vi "Assign values from string to axes_C-887.vi"(0 "System no.":i32=1 min=1 max=4 step=1, 2 "Queried axes":string[](array[string]), 3 "All axes queried?":bool, 4 "Input String":string, 5 "error in":errorcluster, 6 "Axes related?":bool=TRUE) -> (14 "Values":dbl[](array[numeric]) format="%.6f", 15 "Strings":string[](array[string]), 16 "Queried axes out":string[](array[string]), 19 "error out":errorcluster)   [LabVIEW 2020]
doc: "This VI assigns numerical values and/or single lines from input string to queried axes. If All axes is TRUE, connected axes are read from Global2.vi and displayed on the front panel for assignment."
panel:
  # "This vi assigns values and/or single lines from input string to queried axes. If \"All axes\" is true, connected axes are read from Global2.vi"
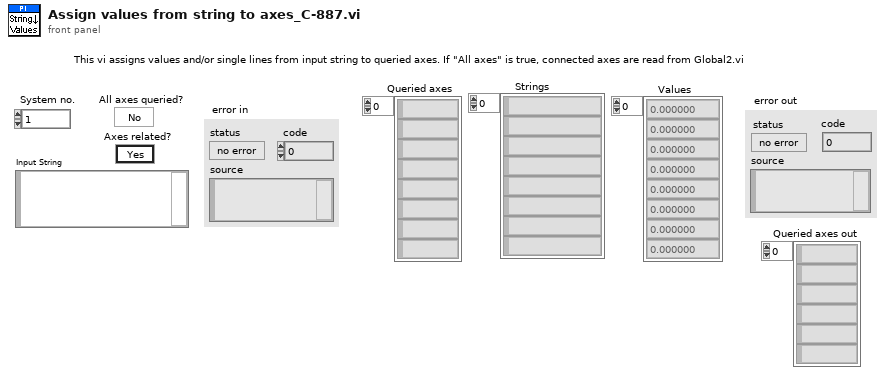
[diagram p1: front panel]
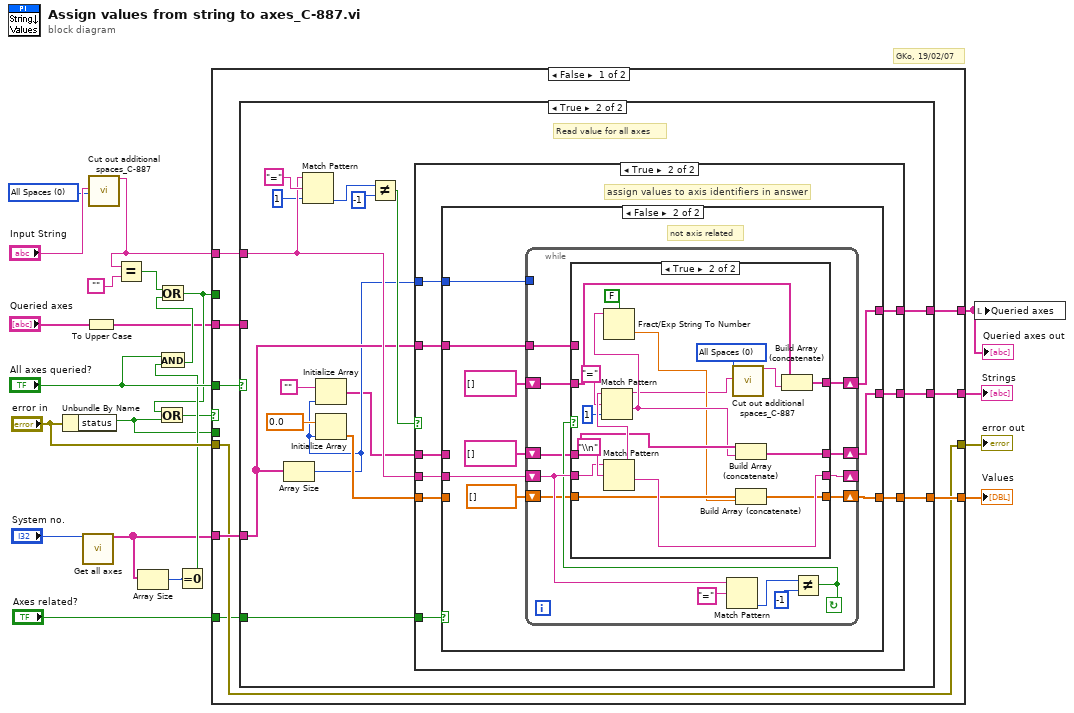
[diagram p0: block diagram]
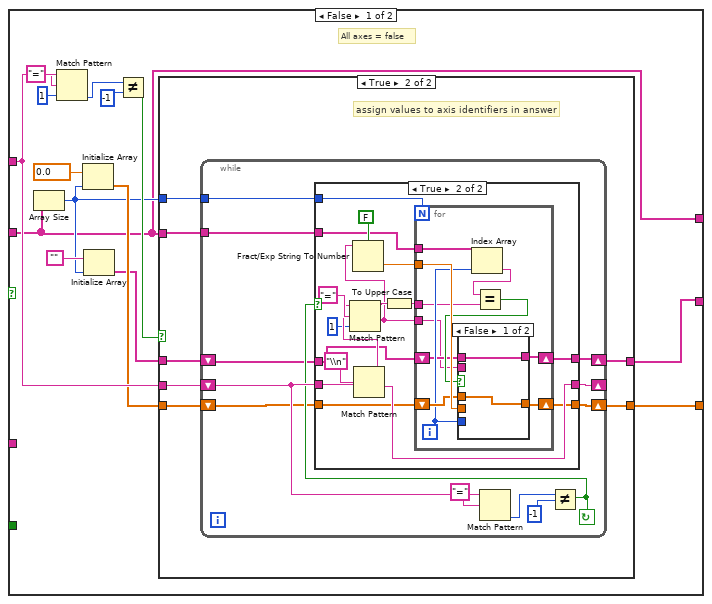
[diagram p2: hidden frame]
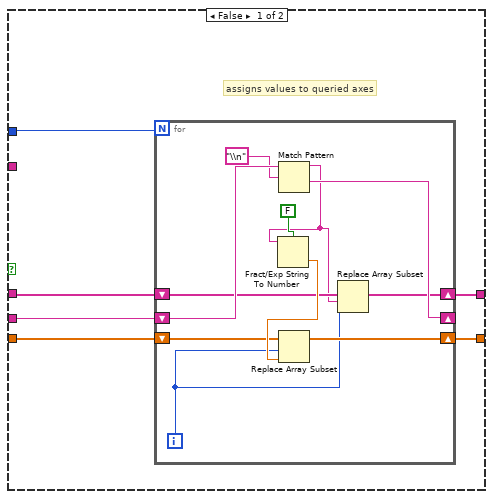
[diagram p3: hidden frame]
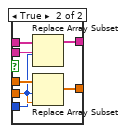
[diagram p5: hidden frame]
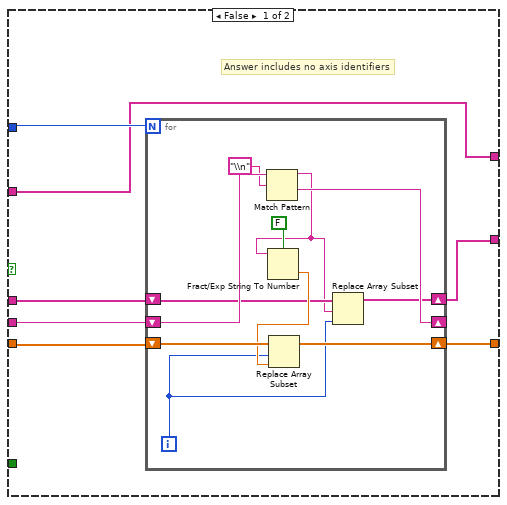
[diagram p6: hidden frame]
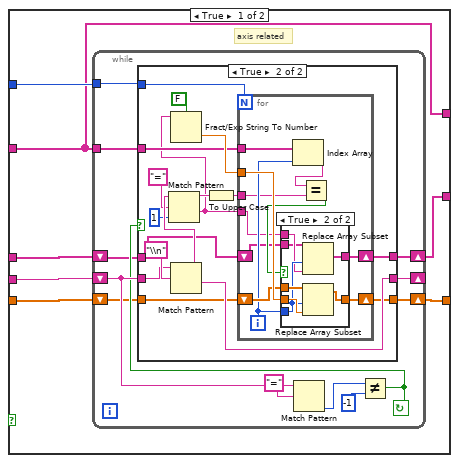
[diagram p7: hidden frame]
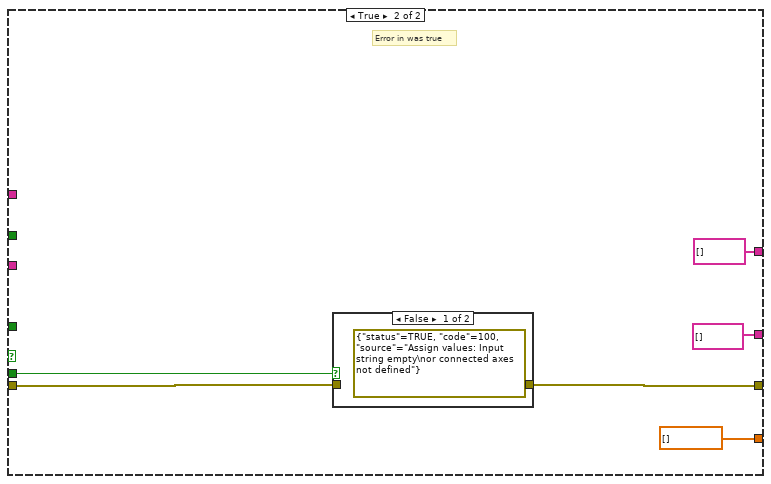
[diagram p11: hidden frame]
diagram:
  w4 = u16 0 items=["All Spaces", "Only if 1st char.", "Only if last char.", "Only if near \"=\""] ("Mode")
  # "GKo, 19/02/07"
  n1 = Unbundle By Name("error in") -> ("status"=w8:bool)
  n2 = call "Get all axes.vi"("System no."="System no.") -> ("Conn. Axes"=w6:string[])  [unwired: 18 out]
  n3 = To Upper Case(1:"Queried axes") -> (0:w10:string[])
  n4 = call "Cut out additional spaces_C-887.vi"("String"="Input String", "Mode"=w4) -> ("String out"=w3:string)  [unwired: 17 out]
  n5 = Equal?(x=w3, y="") -> (x = y?=w17:bool)
  n6 = Array Size(array=w6) -> (size(s)=w15:i32)
  n7 = Equal To 0?(x=w15) -> (x = 0?=w14:bool)
  n8 = And(x="All axes queried?", y=w14) -> (x .and. y?=w13:bool)
  n9 = Or(x=w17, y=w13) -> (x .or. y?=w11:bool)
  n10 = Or(x=w11, y=w8) -> (x .or. y?=w12:bool)
  n11 = case shown="False" w12 {
    tunnel: "All axes queried?" -> [w31 _]
    tunnel: w3 -> [w30 _]
    tunnel: [w29 dbl[] [] ("Step Size")] -> w22
    tunnel: w10 -> [w28 _]
    tunnel: w6 -> [w27 _]
    tunnel: [w26 w271] -> w19
    tunnel: "error in" -> [w26 w272]
    tunnel: w11 -> [_ _]
    tunnel: [w25 string[] []] -> w9
    tunnel: w8 -> [_ w269]
    tunnel: "Axes related?" -> [w24 _]
    tunnel: [w23 string[] [] ("Conn. Axes")] -> w1
    frame False {
      n12 = case shown="True" w31 {
        tunnel: w30 -> [w44 w133]
        tunnel: [w45 w137] -> w29
        tunnel: w28 -> [w32 _]
        tunnel: w27 -> [_ w129]
        tunnel: [w34 w125] -> w25
        tunnel: w24 -> [_ w123]
        tunnel: [w32 w122] -> w23
        frame False {
          # "All axes = false"
          n13 = Array Size(array=w32) -> (size(s)=w36:i32)
          n14 = Match Pattern(string=w44, regular expression="=", offset (0)=1) -> (offset past match=w41:i32)  [unwired: 3 out]
          n15 = Initialize Array(0.0 ("Element Data"), w36) -> (w38:dbl[])
          n16 = Initialize Array("", w36) -> (w35:string[])
          n17 = Not Equal?(x=w41, y=-1) -> (x != y?=w40:bool)
          n18 = case shown="True" w40 {
            tunnel: [w51 w68] -> w45
            tunnel: w44 -> [w50 w69]
            tunnel: w32 -> [_ w67]
            tunnel: w38 -> [w49 w65]
            tunnel: w36 -> [w48 w66]
            tunnel: w35 -> [w47 w64]
            tunnel: [w46 w63] -> w34
            frame False {
              # "assigns values to queried axes"
              n19 = for {
                N: w48 -> [_]
                shift-right: [w56] -> w51
                shift-left: w49 -> [w57]
                shift-right: [w61] -> _
                shift-left: w50 -> [w62]
                shift-right: [w55] -> w46
                shift-left: w47 -> [w54]
                i -> [w53]
                n20 = Match Pattern(string=w62, regular expression="\\n") -> (before substring=w52:string, after substring=w61:string)  [unwired: 3 out]
                n21 = Fract/Exp String To Number(use system decimal point (T)=FALSE, string=w52) -> (number=w58:dbl)  [unwired: 3 out]
                n22 = Replace Array Subset(array=w57, new element=w58, index=w53) -> (w56:dbl[])
                n23 = Replace Array Subset(array=w54, new element=w52, index=w53) -> (w55:string[])
              }
            }
            frame True {
              # "assign values to axis identifiers in answer"
              n24 = while {
                shift-left: w64 -> [w70]
                shift-right: [w71] -> w63
                tunnel: w66 -> [w72]
                tunnel: w67 -> [w73]
                shift-left: w65 -> [w75]
                shift-right: [w74] -> w68
                shift-left: w69 -> [w78]
                shift-right: [w77] -> _
                stop <- w76 continue-if-true
                n25 = Match Pattern(string=w78, regular expression="=") -> (offset past match=w79:i32)  [unwired: 4 out]
                n26 = Not Equal?(x=w79, y=-1) -> (x != y?=w76:bool)
                n27 = case shown="True" w76 {
                  tunnel: w78 -> [w84 w100]
                  tunnel: [w84 w99] -> w77
                  tunnel: [w83 w97] -> w74
                  tunnel: w75 -> [w83 w98]
                  tunnel: w73 -> [_ w92]
                  tunnel: w72 -> [_ w90]
                  tunnel: [w82 w88] -> w71
                  tunnel: w70 -> [w82 w87]
                  frame False {
                  }
                  frame True {
                    n28 = Match Pattern(string=w100, regular expression="\\n") -> (before substring=w94:string, after substring=w99:string)  [unwired: 3 out]
                    n29 = Match Pattern(string=w94, regular expression="=", offset (0)=1) -> (before substring=w91:string, after substring=w89:string)  [unwired: 2 out]
                    n30 = Fract/Exp String To Number(use system decimal point (T)=FALSE, string=w89) -> (number=w93:dbl)  [unwired: 3 out]
                    n31 = To Upper Case(1:w91) -> (0:w85:string)
                    n32 = for {
                      N: w90 -> [_]
                      tunnel: w93 -> [w112]
                      shift-right: [w110] -> w97
                      shift-left: w98 -> [w111]
                      tunnel: w92 -> [w108]
                      tunnel: w85 -> [w106]
                      shift-right: [w103] -> w88
                      shift-left: w87 -> [w104]
                      tunnel: w89 -> [w102]
                      i -> [w109]
                      n33 = Index Array(array=w108, index=w109) -> (element=w107:string)
                      n34 = Equal?(x=w107, y=w106) -> (x = y?=w105:bool)
                      n35 = case shown="False" w105 {
                        tunnel: w112 -> [_ w121]
                        tunnel: w109 -> [_ w118]
                        tunnel: w111 -> [w114 w120]
                        tunnel: [w114 w119] -> w110
                        tunnel: w104 -> [w113 w117]
                        tunnel: [w113 w116] -> w103
                        tunnel: w102 -> [_ w115]
                        frame False {
                        }
                        frame True {
                          n36 = Replace Array Subset(array=w117, new element=w115, index=w118) -> (w116:string[])
                          n37 = Replace Array Subset(array=w120, new element=w121, index=w118) -> (w119:dbl[])
                        }
                      }
                    }
                  }
                }
              }
            }
          }
        }
        frame True {
          # "Read value for all axes"
          n38 = Array Size(array=w129) -> (size(s)=w128:i32)
          n39 = Match Pattern(string=w133, regular expression="=", offset (0)=1) -> (offset past match=w134:i32)  [unwired: 3 out]
          n40 = Initialize Array("", w128) -> (w127:string[])
          n41 = Initialize Array(0.0 ("Element Data"), w128) -> (w130:dbl[])
          n42 = Not Equal?(x=w134, y=-1) -> (x != y?=w132:bool)
          n43 = case shown="True" w132 {
            tunnel: [w144 w164] -> w137
            tunnel: w133 -> [w143 w163]
            tunnel: w129 -> [w138 w162]
            tunnel: w130 -> [w142 w161]
            tunnel: w128 -> [w141 w160]
            tunnel: w127 -> [w140 w159]
            tunnel: [w139 w158] -> w125
            tunnel: w123 -> [_ w157]
            tunnel: [w138 w156] -> w122
            frame False {
              # "Answer includes no axis identifiers"
              n44 = for {
                N: w141 -> [_]
                shift-right: [w151] -> w144
                shift-left: w142 -> [w153]
                shift-right: [w154] -> _
                shift-left: w143 -> [w155]
                shift-right: [w146] -> w139
                shift-left: w140 -> [w148]
                i -> [w147]
                n45 = Match Pattern(string=w155, regular expression="\\n") -> (before substring=w145:string, after substring=w154:string)  [unwired: 3 out]
                n46 = Fract/Exp String To Number(use system decimal point (T)=FALSE, string=w145) -> (number=w152:dbl)  [unwired: 3 out]
                n47 = Replace Array Subset(array=w153, new element=w152, index=w147) -> (w151:dbl[])
                n48 = Replace Array Subset(array=w148, new element=w145, index=w147) -> (w146:string[])
              }
            }
            frame True {
              # "assign values to axis identifiers in answer"
              n49 = case shown="False" w157 {
                tunnel: [w171 w232] -> w164
                tunnel: w163 -> [w170 w231]
                tunnel: w162 -> [w165 w230]
                tunnel: w161 -> [w169 _]
                tunnel: w160 -> [w168 w229]
                tunnel: w159 -> [w167 _]
                tunnel: [w166 w228] -> w158
                tunnel: [w165 w224] -> w156
                frame True {
                  # "axis related"
                  n50 = while {
                    shift-left: w167 -> [w173]
                    shift-right: [w172] -> w166
                    tunnel: w168 -> [w174]
                    tunnel: w165 -> [w175]
                    shift-left: w169 -> [w177]
                    shift-right: [w176] -> w171
                    shift-left: w170 -> [w180]
                    shift-right: [w179] -> _
                    stop <- w178 continue-if-true
                    n51 = Match Pattern(string=w180, regular expression="=") -> (offset past match=w181:i32)  [unwired: 4 out]
                    n52 = Not Equal?(x=w181, y=-1) -> (x != y?=w178:bool)
                    n53 = case shown="True" w178 {
                      tunnel: w180 -> [w186 w202]
                      tunnel: [w186 w201] -> w179
                      tunnel: [w185 w199] -> w176
                      tunnel: w177 -> [w185 w200]
                      tunnel: w175 -> [_ w193]
                      tunnel: w174 -> [_ w192]
                      tunnel: w173 -> [w184 w191]
                      tunnel: [w184 w190] -> w172
                      frame False {
                      }
                      frame True {
                        n54 = Match Pattern(string=w202, regular expression="\\n") -> (before substring=w198:string, after substring=w201:string)  [unwired: 3 out]
                        n55 = Match Pattern(string=w198, regular expression="=", offset (0)=1) -> (before substring=w196:string, after substring=w189:string)  [unwired: 2 out]
                        n56 = Fract/Exp String To Number(use system decimal point (T)=FALSE, string=w189) -> (number=w195:dbl)  [unwired: 3 out]
                        n57 = To Upper Case(1:w196) -> (0:w187:string)
                        n58 = for {
                          N: w192 -> [_]
                          tunnel: w187 -> [w208]
                          tunnel: w195 -> [w214]
                          shift-right: [w212] -> w199
                          shift-left: w200 -> [w213]
                          tunnel: w193 -> [w211]
                          shift-right: [w206] -> w190
                          shift-left: w191 -> [w204]
                          tunnel: w189 -> [w205]
                          i -> [w210]
                          n59 = Index Array(array=w211, index=w210) -> (element=w209:string)
                          n60 = Equal?(x=w209, y=w208) -> (x = y?=w207:bool)
                          n61 = case shown="True" w207 {
                            tunnel: w214 -> [_ w223]
                            tunnel: w210 -> [_ w220]
                            tunnel: w213 -> [w216 w222]
                            tunnel: [w216 w221] -> w212
                            tunnel: [w215 w219] -> w206
                            tunnel: w205 -> [_ w218]
                            tunnel: w204 -> [w215 w217]
                            frame False {
                            }
                            frame True {
                              n62 = Replace Array Subset(array=w217, new element=w218, index=w220) -> (w219:string[])
                              n63 = Replace Array Subset(array=w222, new element=w223, index=w220) -> (w221:dbl[])
                            }
                          }
                        }
                      }
                    }
                  }
                }
                frame False {
                  # "not axis related"
                  n64 = while {
                    shift-left: string[] [] -> [w236]
                    shift-right: [w235] -> w228
                    tunnel: w229 -> [_]
                    tunnel: w230 -> [w237]
                    shift-left: dbl[] [] -> [w239]
                    shift-right: [w238] -> w232
                    shift-left: w231 -> [w242]
                    shift-right: [w241] -> _
                    shift-right: [w234] -> w224
                    shift-left: string[] [] -> [w233]
                    stop <- w240 continue-if-true
                    n65 = Match Pattern(string=w242, regular expression="=") -> (offset past match=w243:i32)  [unwired: 4 out]
                    n66 = Not Equal?(x=w243, y=-1) -> (x != y?=w240:bool)
                    n67 = case shown="True" w240 {
                      tunnel: w242 -> [w249 w266]
                      tunnel: [w249 w265] -> w241
                      tunnel: [w248 w263] -> w238
                      tunnel: w239 -> [w248 w264]
                      tunnel: w237 -> [_ _]
                      tunnel: w236 -> [w247 w259]
                      tunnel: [w247 w258] -> w235
                      tunnel: [w246 w251] -> w234
                      tunnel: w233 -> [w246 w250]
                      frame False {
                      }
                      frame True {
                        w253 = u16 0 items=["All Spaces", "Only if 1st char.", "Only if last char.", "Only if near \"=\"", "Only if 1st or last char.", "Only multiple", "Really all"] ("Mode")
                        n68 = Match Pattern(string=w266, regular expression="\\n") -> (before substring=w262:string, after substring=w265:string)  [unwired: 3 out]
                        n69 = Match Pattern(string=w262, regular expression="=", offset (0)=1) -> (before substring=w254:string, after substring=w256:string)  [unwired: 2 out]
                        n70 = Fract/Exp String To Number(use system decimal point (T)=FALSE, string=w256) -> (number=w255:dbl)  [unwired: 3 out]
                        n71 = call "Cut out additional spaces_C-887.vi"("String"=w254, "Mode"=w253) -> ("String out"=w252:string)  [unwired: 17 out]
                        n72 = Build Array (concatenate)(w259, w256) -> (w258:string[])
                        n73 = Build Array (concatenate)(w264, w255) -> (w263:dbl[])
                        n74 = Build Array (concatenate)(w250, w252) -> (w251:string[])
                      }
                    }
                  }
                }
              }
            }
          }
        }
      }
    }
    frame True {
      # "Error in was true"
      n75 = case shown="False" w269 {
        tunnel: w272 -> [_ w275]
        tunnel: [errorcluster {"status"=TRUE, "code"=100, "source"="Assign values: Input string empty\nor connected axes not defined"} ("error out") w275] -> w271
        frame False {
        }
        frame True {
        }
      }
    }
  }
  "Values" <- w22
  "error out" <- w19
  "Strings" <- w9
  "Queried axes out" <- w1
  n76 = local write "Queried axes"(w1) -> ()
